vi "SFOAE-Initialize Data Processing.vi"(0 "SFOAE":T3, 1 "nfft":i32, 2 "offset":i32, 3 "StimLen":i32, 5 "State":T1, 7 "StimMagRef":refnum<vi>, 9 "OAEMagRef":refnum<vi>, 11 "error in":errorcluster, 12 "OAEPhsRef":refnum<vi>) -> (6 "Expt State out":T1, 10 "DataProc":T2, 15 "error out":errorcluster)   [LabVIEW 2020]
uses:
  Typedefs/SFOAE-Parameters.ctl
  Typedefs/SFOAE-Stimulus Parameters.ctl
  Typedefs/SFOAE-Sweep Params.ctl
  Typedefs/SFOAE-Response Parameters.ctl
  CFTS Main Panel SubVIs/CFTS-Experiment State.ctl
  Typedefs/SFOAE-Data Processing.ctl
  epl-vi-lib/Utility VIs/Math VIs/dB to Linear (scalar).vi
  epl-vi-lib/Utility VIs/Math VIs/Linear to dB (scalar).vi
  epl-vi-lib/Utility VIs/Math VIs/LinSpace (start-stop-step).vi
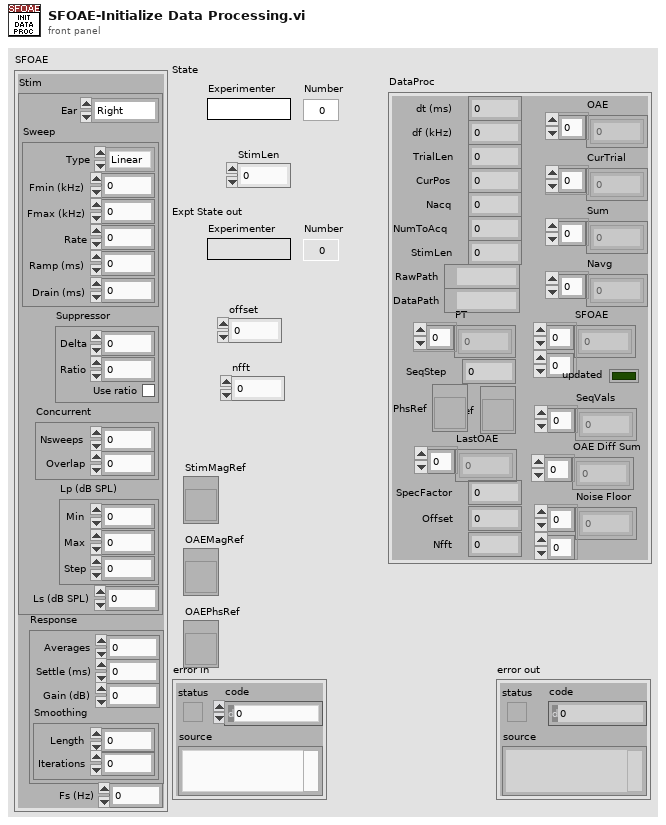
[diagram p1: front panel]
types:
  T1 = typedef "CFTS-Experiment State.ctl" = cluster{"Experimenter":string, "Number":u32, "Right":string, "Left":string, "Data Folder":path, "State File":path, "Version Info":string, "End Exposure Time":dbl, "Exposure Duration":string, "Run #":cluster{"CAP":i16, "ABR":i16, "DP":i16, "VsEP":i16, "MeasSeq":i16, "SubSeq":i16, "SFOAE":i16}}
  T2 = typedef "SFOAE-Data Processing.ctl" = cluster{"dt (ms)":dbl, "TrialLen":i32, "PT":cdb[], "CurPos":i32, "Sum":dbl[], "Navg":dbl[], "Nacq":i32, "RawPath":path, "DataPath":path, "NumToAcq":i32, "OAE":dbl[], "CurTrial":dbl[], "StimLen":i32, "SFOAE":cdb[][], "SeqStep":i32, "updated":bool, "SeqVals":dbl[], "df (kHz)":dbl, "MagRef":refnum<vi>, "LastOAE":dbl[], "OAE Diff Sum":dbl[], "Noise Floor":cdb[][], "SpecFactor":dbl, "Offset":i32, "Nfft":i32, "PhsRef":refnum<vi>}
  T3 = typedef "SFOAE-Parameters.ctl" = cluster{"Stim":T4, "Response":T6, "Fs (Hz)":dbl}
  T4 = typedef "SFOAE-Stimulus Parameters.ctl" = cluster{"Ear":enum16{"Right", "Left"}, "Sweep":T5, "Suppressor":cluster{"Delta":dbl, "Ratio":dbl, "Use ratio":bool}, "Concurrent":cluster{"Nsweeps":i32, "Overlap":dbl}, "Ls (dB SPL)":dbl, "Lp (dB SPL)":cluster{"Min":dbl, "Max":dbl, "Step":dbl}}
  T5 = typedef "SFOAE-Sweep Params.ctl" = cluster{"Type":enum16{"Linear", "Log"}, "Fmin (kHz)":dbl, "Fmax (kHz)":dbl, "Rate":dbl, "Ramp (ms)":dbl, "Drain (ms)":dbl}
  T6 = typedef "SFOAE-Response Parameters.ctl" = cluster{"Averages":i32, "Settle (ms)":dbl, "Gain (dB)":dbl, "Smoothing":cluster{"Length":i32, "Iterations":i32}}
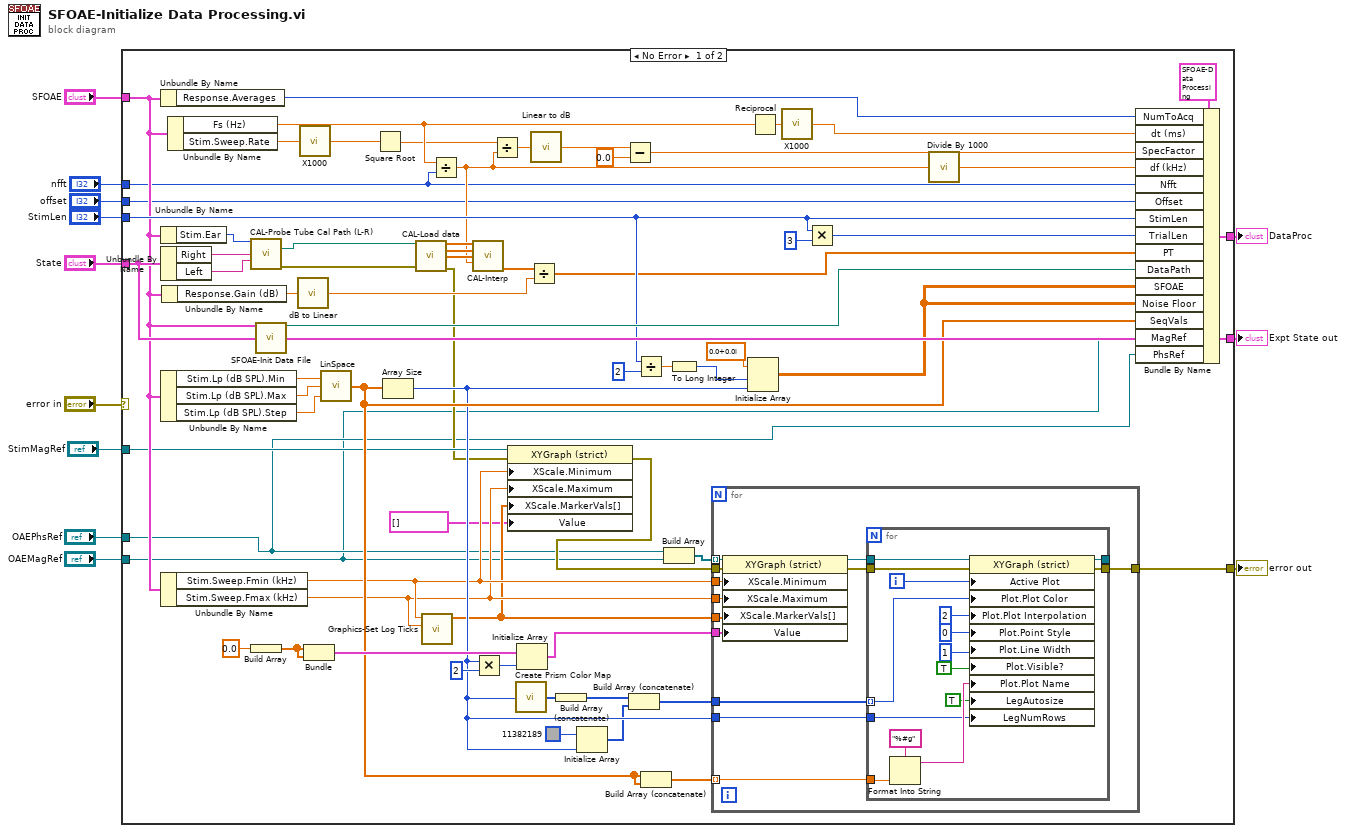
[diagram p0: block diagram]
diagram:
  n1 = case shown="No Error" "error in" {
    selector: "error in" -> [_ w109]
    tunnel: [w80 _] -> w12
    tunnel: [w77 w110] -> w11
    tunnel: "SFOAE" -> [w46 _]
    tunnel: "State" -> [w53 w110]
    tunnel: "StimLen" -> [w52 _]
    tunnel: "OAEMagRef" -> [w13 _]
    tunnel: [w48 w109] -> w5
    tunnel: "StimMagRef" -> [w26 _]
    tunnel: "nfft" -> [w17 _]
    tunnel: "offset" -> [w16 _]
    tunnel: "OAEPhsRef" -> [w14 _]
    frame No Error {
      n2 = Unbundle By Name(w46) -> ("Response.Averages"=w76:i32)
      n3 = Unbundle By Name(w46) -> ("Stim.Ear"=w67:enum16{"Right", "Left"})
      n4 = Unbundle By Name(w53) -> ("Right"=w74:string, "Left"=w73:string)
      n5 = Unbundle By Name(w46) -> ("Stim.Lp (dB SPL).Min"=w62:dbl, "Stim.Lp (dB SPL).Max"=w61:dbl, "Stim.Lp (dB SPL).Step"=w60:dbl)
      n6 = Unbundle By Name(w46) -> ("Stim.Sweep.Fmin (kHz)"=w25:dbl, "Stim.Sweep.Fmax (kHz)"=w24:dbl)
      n7 = Unbundle By Name(w46) -> ("Response.Gain (dB)"=w45:dbl)
      n8 = Unbundle By Name(w46) -> ("Fs (Hz)"=w49:dbl, "Stim.Sweep.Rate"=w32:dbl)
      n9 = call "CAL-Probe Tube Cal Path (L-R).vi"("Ear"=w67, "Right"=w74, "Left"=w73) -> ("Probe Tube Cal Path"=w71:path, "error out"=w72:errorcluster)  [unwired: 11 in]
      n10 = Build Array(0.0) -> (w58:dbl[])
      n11 = call "SFOAE-Init Data File.vi"("SFOAE"=w46, "State"=w53) -> ("DataPath"=w78:path, "Expt State out"=w77:T1)  [unwired: 12 in]
      n12 = call-poly "dB to Linear.vi"("dB"=w45) -> ("linear"=w43:dbl)
      n13 = call "X1000.vi"("X"=w32) -> ("X/1000"=w27:dbl)
      n14 = Bundle(w58, w58) -> (w57:cluster{dbl[], dbl[]})  [unwired: 1 in]
      n15 = call-poly "LinSpace.vi"("Step"=w60, "Stop"=w61, "Start"=w62) -> ("Array"=w37:dbl[])  [unwired: 1 in, 1 out]
      n16 = Square Root(x=w27) -> (sqrt(x)=w31:dbl)
      n17 = Array Size(array=w37) -> (size(s)=w35:i32)
      n18 = call "CAL-Load data.vi"("user path"=w71, "error in (no error)"=w72) -> ("Frequency (Hz)"=w70:dbl[], "Mag"=w69:dbl[], "Phase"=w68:dbl[], "error out"=w22:errorcluster)  [unwired: 6 in, 4 out]
      n19 = call "Graphics-Set Log Ticks.vi"("Max"=w24, "Min"=w25) -> ("Tick Vals"=w23:dbl[])  [unwired: 9 in]
      n20 = Divide(x=w49, y=w17) -> (x/y=w30:dbl)
      n21 = call "CAL-Interp.vi"("Frequency (Hz)"=w70, "Magnitude (dB)"=w69, "Phase (degrees)"=w68, "df (Hz)"=w30) -> ("Interp z"=w47:cdb[])  [unwired: 8 in, 3 out]
      n22 = Multiply(x=w35, y=2) -> (x*y=w39:i32)
      n23 = Divide(x=w31, y=w30) -> (x/y=w29:dbl)
      n24 = property on="Property Node" class="XYGraph (strict)"(reference=w26, error in=w22, "XScale.Minimum"=w25, "XScale.Maximum"=w24, "XScale.MarkerVals[]"=w23, "Value"=cluster{"Array":dbl[], "Array":dbl[]}[] []) -> (error out=w21:errorcluster)  [unwired: 1 out]
      n25 = call "Create Prism Color Map.vi"("Size"=w35) -> ("Colors"=w55:u32[])
      n26 = Initialize Array(w57, w39) -> (w56:cluster{dbl[], dbl[]}[])
      n27 = Divide(x=w47, y=w43) -> (x/y=w44:cdb[])
      n28 = call-poly "Linear to dB.vi"("Linear"=w29) -> ("dB"=w28:dbl)
      n29 = Build Array (concatenate)(w55) -> (w54:u32[])
      n30 = Initialize Array(u32 11382189, w35) -> (w33:u32[])
      n31 = Subtract(x=w28, y=0.0) -> (x-y=w19:dbl)
      n32 = Build Array (concatenate)(w54, w33) -> (w36:u32[])
      n33 = Divide(x=w52, y=2) -> (x/y=w65:dbl)
      n34 = Build Array (concatenate)(w37, w37) -> (w38:dbl[])
      n35 = Build Array(w14, w13) -> (w15:refnum<vi>[])
      n36 = To Long Integer(number=w65) -> (32bit integer=w63:i32)
      n37 = for {
        tunnel: w56 -> [w93]
        tunnel: w15 -> [w91] mode=indexing
        tunnel: [w89] -> w48
        tunnel: w38 -> [w88] mode=indexing
        tunnel: w36 -> [w87]
        tunnel: w35 -> [w86]
        tunnel: w25 -> [w85]
        tunnel: w24 -> [w84]
        tunnel: w23 -> [w83]
        tunnel: w21 -> [w82]
        n38 = property on="Property Node" class="XYGraph (strict)"(reference=w91, error in=w82, "XScale.Minimum"=w85, "XScale.Maximum"=w84, "XScale.MarkerVals[]"=w83, "Value"=w93) -> (reference out=w90:refnum<vi>, error out=w92:errorcluster)
        n39 = for {
          tunnel: w87 -> [w101] mode=indexing
          tunnel: w92 -> [w108]
          tunnel: w88 -> [w103]
          tunnel: w90 -> [w98]
          tunnel: [w97] -> w89
          tunnel: [w96] -> _
          tunnel: w86 -> [w94]
          i -> [w102]
          n40 = Format Into String(format string="%#g", w103) -> (resulting string=w99:string)  [unwired: 2 in, 1 out]
          n41 = property on="Property Node" class="XYGraph (strict)"(reference=w98, error in=w108, "Active Plot"=w102, "Plot.Plot Color"=w101, "Plot.Plot Interpolation"=u8 2, "Plot.Point Style"=u8 0, "Plot.Line Width"=u8 1, "Plot.Visible?"=TRUE ("Plot.Visible"), "Plot.Plot Name"=w99, "LegAutosize"=TRUE ("Legend:Autosize"), "LegNumRows"=w94) -> (reference out=w96:refnum<vi>, error out=w97:errorcluster)
        }
      }
      n42 = Initialize Array(cdb 0.0+0.0i ("element"), w63, w35) -> (w41:cdb[][])
      n43 = Reciprocal(x=w49) -> (1/x=w50:dbl)
      n44 = call "X1000.vi"("X"=w50) -> ("X/1000"=w51:dbl)
      n45 = Multiply(x=w52, y=3) -> (x*y=w75:i32)
      n46 = call "Divide By 1000.vi"("X"=w30) -> ("X/1000"=w42:dbl)
      n47 = Bundle By Name(cluster=T2 {"dt (ms)"=0.0, "TrialLen"=0, "PT"=[], "CurPos"=0, "Sum"=[], "Navg"=[], "Nacq"=0, "RawPath"=path "", "DataPath"=path "", "NumToAcq"=0, "OAE"=[], "CurTrial"=[], "StimLen"=0, "SFOAE"=[], "SeqStep"=0, "updated"=FALSE, "SeqVals"=[], "df (kHz)"=0.0, "MagRef"=refnum, "LastOAE"=[], "OAE Diff Sum"=[], "Noise Floor"=[], "SpecFactor"=0.0, "Offset"=0, "Nfft"=0, "PhsRef"=refnum} ("DataProc"), "NumToAcq"=w76, "dt (ms)"=w51, "SpecFactor"=w19, "df (kHz)"=w42, "Nfft"=w17, "Offset"=w16, "StimLen"=w52, "TrialLen"=w75, "PT"=w44, "DataPath"=w78, "SFOAE"=w41, "Noise Floor"=w41, "SeqVals"=w37, "MagRef"=w13, "PhsRef"=w14) -> (w80:T2)
    }
    frame Error {
    }
  }
  "error out" <- w5
  "DataProc" <- w12
  "Expt State out" <- w11
